vi "DIO64 Out Config.vi"(0 "board in":u16 format="%.0x", 1 "#ports":u8=1 min=1 max=8, 2 "divider":u32 min=1 max=8, 5 "scan rate (Hz)":dbl=10000.0 format="%.2f", 7 "mask":u16[](array[numeric])=[1] format="%.0x", 9 "Config Control":T1 {"#transitions" format="%.0x"; "repetitions" format="%.0x"; "DAQ clock modulo" format="%.0x"}, 11 "error in (no error)":errorcluster) -> (4 "board out":u16 format="%.0x", 6 "actual scan rate (Hz)":dbl=10000.0 format="%.2f", 15 "error out":errorcluster)   [LabVIEW 2012]
doc: "DIO64 Out Config establishes the parameters for an output operation on the digital I/O board. This must be performed before data is written or the output operation is started. \n\nNote: This VI is only used for output-only and combined input and output board modes. This VI will generate an error in input-only board mode.\n\n\nCopyright (c) 2002 Viewpoint Systems Inc. All Rights Reserved\n\nadded missing divider control"
uses:
  DIO64 Out Config Control.ctl
  DIO64 Clock Control.ctl
  DIO64 Start Trig.ctl
  DIO64 Stop Trig.ctl
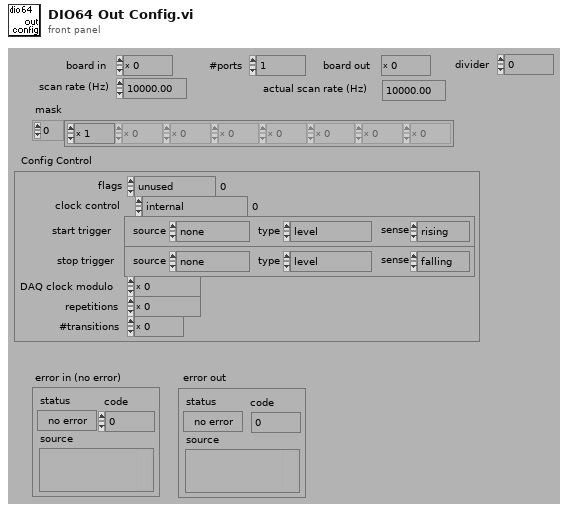
[diagram p1: front panel]
types:
  T1 = typedef "DIO64 Out Config Control.ctl" = cluster{"flags":enum16{"unused"}, "clock control":T2, "start trigger":T3, "stop trigger":T4, "DAQ clock modulo":u32, "repetitions":u32, "#transitions":u16}
  T2 = typedef "DIO64 Clock Control.ctl" = enum16{"internal", "external", "trig 0", "OCXO"}
  T3 = typedef "DIO64 start trig.ctl" = cluster{"source":enum16{"none", "internal", "external", "trig 2", "PXI Star"}, "type":enum16{"level", "edge", "edge to edge"}, "sense":enum16{"rising", "falling"}}
  T4 = typedef "DIO64 stop trig.ctl" = cluster{"source":enum16{"none", "internal", "external", "trig 3 in", "output FIFO"}, "type":enum16{"level", "edge"}, "sense":enum16{"falling", "rising"}}
  T5 = enum16{"none", "internal", "external", "trig 3 in", "output FIFO"}
  T6 = enum16{"none", "internal", "external", "trig 2", "PXI Star"}
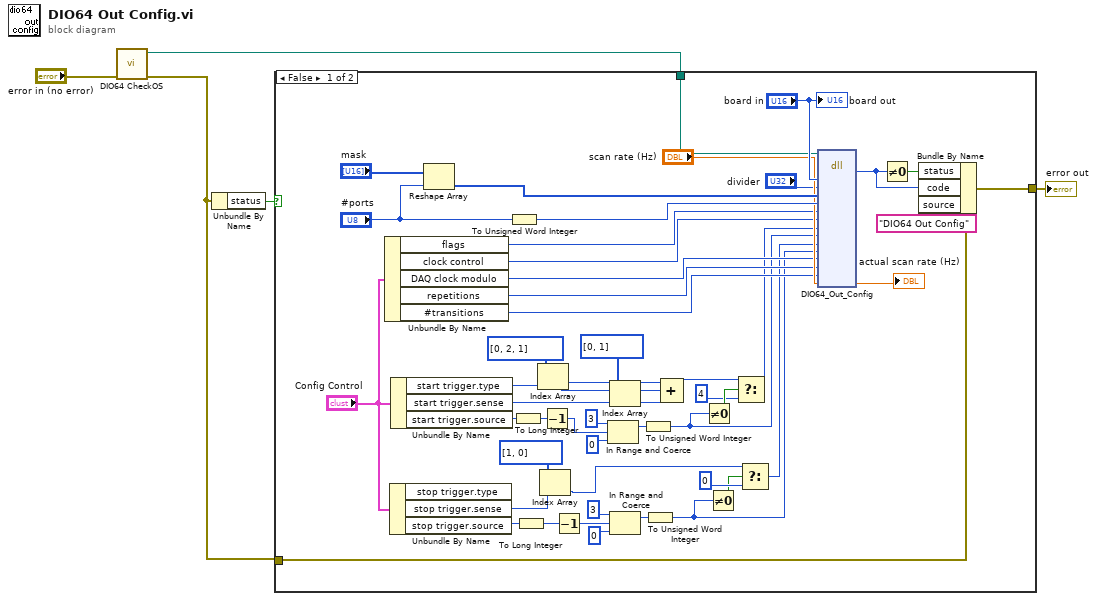
[diagram p0: block diagram]
diagram:
  n1 = call "DIO64 CheckOS.vi"("error in"="error in (no error)") -> ("error out"=w1:errorcluster, "path in"=w3:path)  [unwired: 9 in]
  n2 = Unbundle By Name(w1) -> ("status"=w5:bool)
  n3 = case shown="False" w5 {
    tunnel: w1 -> [w55 w56]
    tunnel: [w52 w56] -> w4
    tunnel: w3 -> [w6 _]
    frame False {
      n4 = Unbundle By Name("Config Control") -> ("flags"=w28:enum16{"unused"}, "clock control"=w27:T2, "DAQ clock modulo"=w26:u32, "repetitions"=w25:u32, "#transitions"=w24:u16)
      n5 = Unbundle By Name("Config Control") -> ("stop trigger.sense"=w20:enum16{"falling", "rising"}, "stop trigger.source"=w31:T5)  [unwired: 1 out]
      n6 = Unbundle By Name("Config Control") -> ("start trigger.type"=w37:enum16{"level", "edge", "edge to edge"}, "start trigger.sense"=w23:enum16{"rising", "falling"}, "start trigger.source"=w39:T6)
      n7 = Reshape Array("mask", "#ports") -> (w50:u16[])
      n8 = To Unsigned Word Integer(number="#ports") -> (unsigned 16bit integer=w47:u16)
      n9 = To Long Integer(number=w39) -> (32bit integer=w14:i32)
      n10 = To Long Integer(number=w31) -> (32bit integer=w13:i32)
      n11 = Index Array(array=u16[] [0, 2, 1], index=w37) -> (element=w36:u16)
      n12 = Index Array(array=u16[] [1, 0], index=w20) -> (element=w9:u16)
      n13 = Decrement(x=w14) -> (x-1=w43:i32)
      n14 = Decrement(x=w13) -> (x-1=w32:i32)
      n15 = In Range and Coerce(upper limit=3 ("lower limit"), x=w43, lower limit=0) -> (coerced(x)=w41:i32)  [unwired: 1 out]
      n16 = Index Array(array=u16[] [0, 1], index=w23) -> (element=w21:u16)
      n17 = In Range and Coerce(upper limit=3 ("lower limit"), x=w32, lower limit=0) -> (coerced(x)=w34:i32)  [unwired: 1 out]
      n18 = To Unsigned Word Integer(number=w41) -> (unsigned 16bit integer=w15:u16)
      n19 = To Unsigned Word Integer(number=w34) -> (unsigned 16bit integer=w10:u16)
      n20 = Compound Arithmetic op=ADD(w36, w36, w21) -> (w16:u16)
      n21 = Not Equal To 0?(x=w15) -> (x != 0?=w19:bool)
      n22 = Not Equal To 0?(x=w10) -> (x != 0?=w11:bool)
      n23 = Select(t=w16, s=w19, f=u16 4) -> (s? t:f=w17:u16)
      n24 = Select(t=w9, s=w11, f=u16 0) -> (s? t:f=w8:u16)
      n25 = dll-call lib="F:/DIO64/Visa_Beta_Feb2014/DIO64Visa_Release Beta 1/DIO64Visa_Release Beta 1/LabVIEW/DIO64_Visa32.dll" fn="DIO64_Out_Config"(path in=w6, "board"="board in", "ticks"="divider", "mask"=w50, "masklength"=w47, "flags"=w28, "clkControl"=w27, "startType"=w17, "startSource"=w15, "stopType"=w8, "stopSource"=w10, "AIControl"=w26, "reps"=w25, "ntrans"=w24, "scanRate"="scan rate (Hz)") -> ("return type"=w53:i32, "scanRate"=→"actual scan rate (Hz)":dbl)  [unwired: 13 in, 4 out]
      n26 = Not Equal To 0?(x=w53) -> (x != 0?=w54:bool)
      n27 = Bundle By Name(cluster=w55, "status"=w54, "code"=w53, "source"="DIO64 Out Config") -> (w52:errorcluster)
      "board out" <- "board in"
    }
    frame True {
    }
  }
  "error out" <- w4
